vi "emi_Is Warning.vi"(14 "error in (no error)":errorcluster) -> (3 "error out":errorcluster, 8 "Is Warning":bool)   [LabVIEW 2010]
doc: "Extracts teh error status from error cluster,\n \n\nSaves Diagram space at teh expence of execution speed."
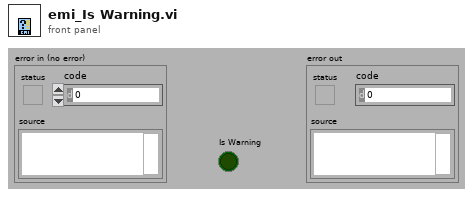
[diagram p1: front panel]
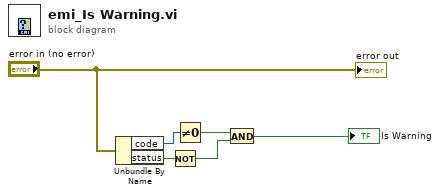
[diagram p0: block diagram]
diagram:
  n1 = Unbundle By Name("error in (no error)") -> ("code"=w6:i32, "status"=w2:bool)
  n2 = Not(x=w2) -> (.not. x?=w5:bool)
  n3 = Not Equal To 0?(x=w6) -> (x != 0?=w4:bool)
  n4 = And(x=w4, y=w5) -> (x .and. y?=→"Is Warning":bool)
  "error out" <- "error in (no error)"
